vi "Add.vi"(8 "error in":errorcluster, 10 "name":string="Ballard ARINC 429", 11 "target in":refnum<k24>) -> (0 "error out":errorcluster, 2 "Ballard ARINC 429 custom device":u64 format="%.0x", 3 "target out":refnum<k24>)   [LabVIEW 2020, in "Ballard ARINC 429 Scripting.lvlib"]
uses:
  NationalInstruments.VeriStand.SystemDefinitionAPI
  Constants.vi
  Ballard ARINC 429 Scripting.lvlib
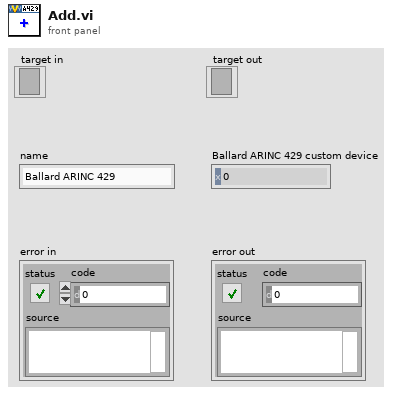
[diagram p1: front panel]
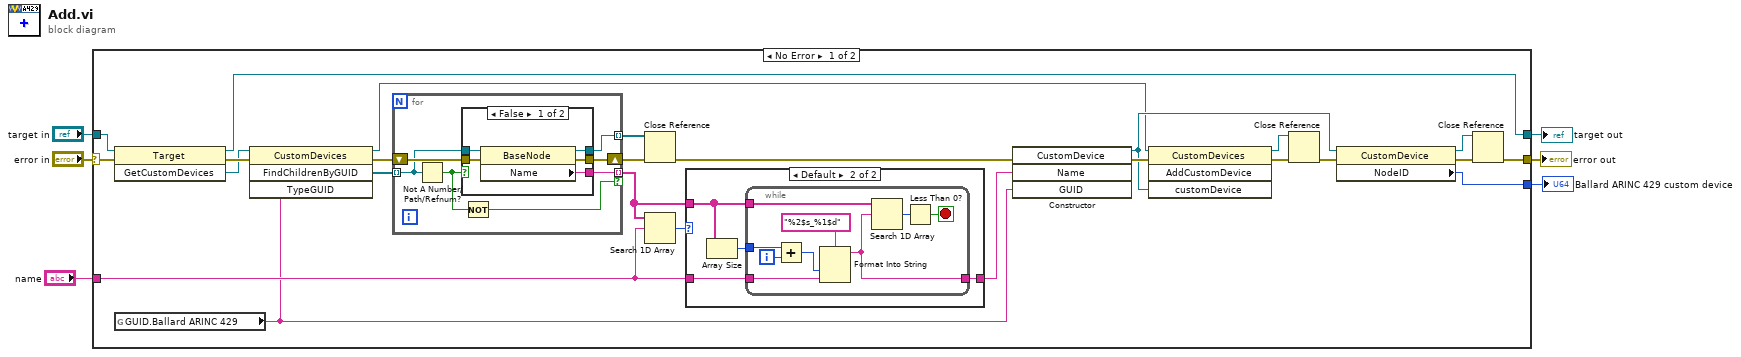
[diagram p0: block diagram]
diagram:
  n1 = case shown="No Error" "error in" {
    selector: "error in" -> [w25 w61]
    tunnel: "target in" -> [w27 w60]
    tunnel: [w19 w61] -> w4
    tunnel: "name" -> [w17 _]
    tunnel: [w10 _] -> w2
    tunnel: [w9 w60] -> w1
    frame No Error {
      n2 = invoke class="Target" method="GetCustomDevices"(reference=w27, error in=w25) -> (reference out=w9:refnum<k24>, error out=w31:errorcluster, "GetCustomDevices"=w30:refnum<k24>)  [unwired: 1 in]
      n3 = global read "Constants.vi" "GUID.Ballard ARINC 429"() -> (w7:string)
      n4 = invoke class="CustomDevices" method="FindChildrenByGUID"(reference=w30, error in=w31, "TypeGUID"=w7) -> (reference out=w14:refnum<k24>, error out=w8:errorcluster, "FindChildrenByGUID"=w26:refnum<k24>[])  [unwired: 1 in, 1 out]
      n5 = for {
        shift-right: [w50] -> w28
        shift-left: w8 -> [w52]
        tunnel: w26 -> [w49] mode=indexing
        tunnel: [w51] -> w29 mode=indexing
        tunnel: [w48] -> w15 mode=indexing if=w46
        n6 = Not A Number/Path/Refnum?(number/path/refnum=w49) -> (NaN/Path/Refnum?=w47:bool)
        n7 = case shown="False" w47 {
          tunnel: [w54 w59] -> w50
          tunnel: w52 -> [w56 w59]
          tunnel: w49 -> [w57 w58]
          tunnel: [w55 w58] -> w51
          tunnel: [w53 _] -> w48
          frame False {
            n8 = property class="BaseNode"(reference=w57, error in=w56) -> (reference out=w55:refnum<k24>, error out=w54:errorcluster, "Name"=w53:string)
          }
          frame True {
          }
        }
        n9 = Not(x=w47) -> (.not. x?=w46:bool)
      }
      n10 = Close Reference(reference=w29, error in (no error)=w28) -> (error out=w20:errorcluster)
      n11 = Search 1D Array(1D array=w15, element=w17) -> (index of element=w18:i32)  [unwired: 1 in]
      n12 = case shown="Default" w18 {
        tunnel: [w32 w33] -> w16
        tunnel: w17 -> [w32 w36]
        tunnel: w15 -> [_ w34]
        frame ..-1 {
        }
        frame Default {
          n13 = Array Size(array=w34) -> (size(s)=w35:i32)
          n14 = while {
            tunnel: w34 -> [w45]
            tunnel: w36 -> [w39]
            tunnel: w35 -> [w42]
            tunnel: [w37] -> w33
            i -> [w41]
            stop <- w43 stop-if-true
            n15 = Add(x=w42, y=w41) -> (x+y=w40:i32)
            n16 = Format Into String(format string="%2$s_%1$d", w40, w39) -> (resulting string=w37:string)  [unwired: 2 in, 1 out]
            n17 = Search 1D Array(1D array=w45, element=w37) -> (index of element=w44:i32)  [unwired: 1 in]
            n18 = Less Than 0?(x=w44) -> (x < 0?=w43:bool)
          }
        }
      }
      n19 = constructor class="CustomDevice"(error in=w20, "Name"=w16, "GUID"=w7) -> (reference out=w21:refnum<k24>, error out=w24:errorcluster)  [unwired: 2 in, 3 out]
      n20 = invoke class="CustomDevices" method="AddCustomDevice"(reference=w14, error in=w24, "customDevice"=w21) -> (reference out=w11:refnum<k24>, error out=w13:errorcluster)  [unwired: 1 in, 2 out]
      n21 = Close Reference(reference=w11, error in (no error)=w13) -> (error out=w12:errorcluster)
      n22 = property class="CustomDevice"(reference=w21, error in=w12) -> (reference out=w23:refnum<k24>, error out=w22:errorcluster, "NodeID"=w10:u64)
      n23 = Close Reference(reference=w23, error in (no error)=w22) -> (error out=w19:errorcluster)
    }
    frame Error {
    }
  }
  "error out" <- w4
  "Ballard ARINC 429 custom device" <- w2
  "target out" <- w1
